vi "Initialization VI.vi"(8 "error in (no error)":errorcluster, 10 "Custom XML":string, 11 "Device Item Ref in":T1 format="%.0x") -> (0 "error out":errorcluster, 3 "Device Item Ref out":T1 format="%.0x")   [LabVIEW 2021, in "Software Multi-Plex System Explorer.lvlib"]
uses:
  Software Multi-Plex System Explorer.lvlib
  <vilib>/NI VeriStand/Custom Device API/Custom Device Item Ref.ctl
  <vilib>/NI/NI VeriStand Custom Device Import and Export Tool/ImportExport.lvlib
  <vilib>/NI VeriStand/Custom Device API/Custom Device API.lvlib
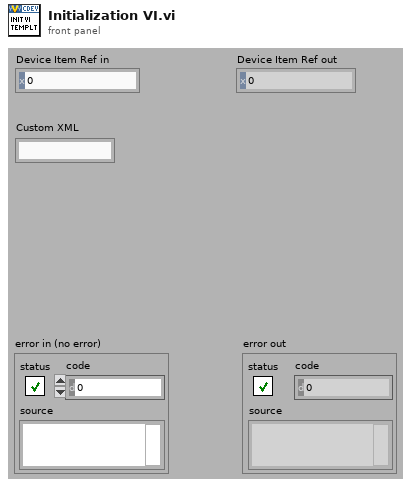
[diagram p1: front panel]
types:
  T1 = typedef "Custom Device API.lvlib/Custom Device Item Ref.ctl" = u64
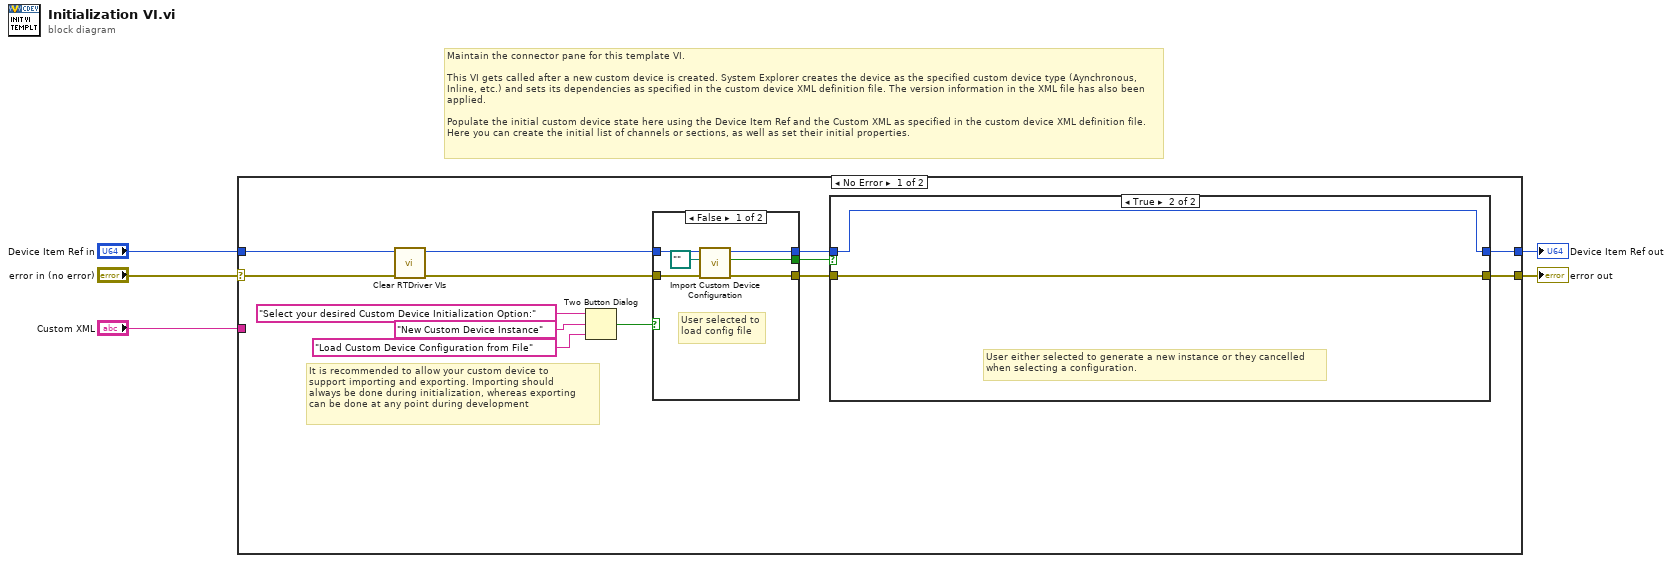
[diagram p0: block diagram]
diagram:
  # "Maintain the connector pane for this template VI.\n\nThis VI gets called after a new custom device is created. System Explorer creates the device as the specified custom device type (Aynchronous, Inline, etc.) and sets its dependencies as specified in the custom device XML definition file. The version information in the XML file has also been applied.\n\nPopulate the initial custom device state here using the Device Item Ref and the Custom XML as specified in the custom device XML definition file. Here you can create the initial list of channels or sections, as well as set their initial properties."
  n1 = case shown="No Error" "error in (no error)" {
    selector: "error in (no error)" -> [w9 w33]
    tunnel: [w11 w33] -> w5
    tunnel: [w10 w32] -> w3
    tunnel: "Device Item Ref in" -> [w8 w32]
    tunnel: "Custom XML" -> [_ _]
    frame No Error {
      # "It is recommended to allow your custom device to\nsupport importing and exporting. Importing should\nalways be done during initialization, whereas exporting\ncan be done at any point during development"
      n2 = call "Clear RTDriver VIs.vi"("error in (no error)"=w9, "Device Item Ref in in"=w8) -> ("error out"=w6:errorcluster, "Device Item Ref out"=w7:T1)  [unwired: 8 in]
      n3 = Two Button Dialog(message="Select your desired Custom Device Initialization Option:", 1:"Load Custom Device Configuration from File" ("F button name (\"Cancel\")"), 2:"New Custom Device Instance" ("T button name (\"OK\")")) -> (T button?=w15:bool)
      n4 = case shown="False" w15 {
        selector: w15 -> [_ w29]
        tunnel: w7 -> [w28 w31]
        tunnel: [w27 w31] -> w14
        tunnel: w6 -> [w25 w30]
        tunnel: [w24 w30] -> w12
        tunnel: [w23 w29] -> w13
        frame False {
          # "User selected to\nload config file"
          n5 = call <vilib>:"Import Custom Device Configuration.vi"("error in (no error)"=w25, "Path"=path "", "NodeID"=w28) -> ("error out"=w24:errorcluster, "cancelled"=w23:bool, "NodeID out"=w27:u64)  [unwired: 6 in]
        }
        frame True {
          # "User selected new\ncustom device. Do\nnothing in this case\nand handle new\ngeneration in the\nnext case structure"
        }
      }
      n6 = case shown="True" w13 {
        tunnel: w14 -> [w20 w22]
        tunnel: w12 -> [w19 w21]
        tunnel: [w19 w21] -> w11
        tunnel: [w20 w22] -> w10
        frame False {
          # "User selected to import from configuration and didn't cancel import"
        }
        frame True {
          # "User either selected to generate a new instance or they cancelled\nwhen selecting a configuration."
        }
      }
    }
    frame Error {
    }
  }
  "error out" <- w5
  "Device Item Ref out" <- w3
